vi "Init Events.vi"(8 "error in (no error)":errorcluster, 11 "LV Chat Server in":refnum<class "LV Chat Server.lvclass">) -> (0 "error out":errorcluster, 3 "LV Chat Server out":refnum<class "LV Chat Server.lvclass">)   [LabVIEW 2020, in "LV Chat Server.lvclass"]
uses:
  LV Chat Server.lvclass
  Stream-Simple-Msg/Endpoint/Endpoint.lvclass
  LV Chat Server.lvclass/LV Chat Server.ctl
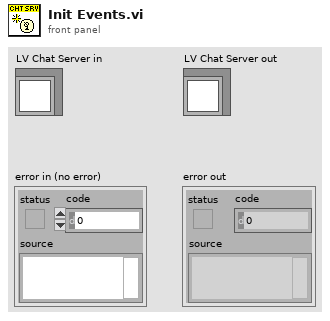
[diagram p1: front panel]
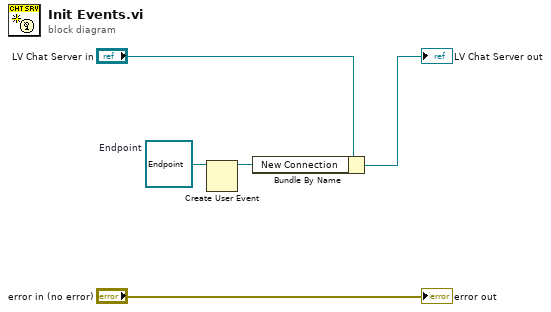
[diagram p0: block diagram]
diagram:
  w2 = refnum<class "Endpoint.lvclass"> refnum  # Endpoint
  n1 = Create User Event(user event datatype=w2) -> (user event=w1:refnum<user-event>)  [unwired: 1 in, 1 out]
  n2 = Bundle By Name(cluster="LV Chat Server in", "New Connection"=w1) -> (→"LV Chat Server out":refnum<class "LV Chat Server.lvclass">)
  "error out" <- "error in (no error)"
